vi "1.Main demo.vi"() -> ()   [LabVIEW 2010]
uses:
  UnderAutomation.Fanuc/UnderAutomation.Fanuc.lvlib
  C:/Users/fg/Documents/Fanuc.vi/LabVIEW_2024/UnderAutomation.Fanuc/lib/UnderAutomation.Fanuc.dll
  LabVIEW_2024/UnderAutomation.Fanuc/lib/UnderAutomation.Fanuc.dll
panel:
  out "CGTP Enabled":bool
  out "Cgtp":refnum<k24>
  out "SNPX connected":bool
  out "FTP connected":bool
  out "Telnet connected":bool
  in  "Tab Control":T1(tab)
  in  "HTTP Password":string caption="HTTP password"
  in  "HTTP Login":string caption="HTTP login (optional)"
  in  "Use CGTP":bool
  in  "Disconnect":bool
  in  "Test":bool
  in  "Key":string
  in  "Licensee":string
  in  "Use SNPX":bool
  in  "FTP password":string
  in  "FTP user":string
  in  "Use FTP":bool
  in  "Connect":bool
  in  "Telnet password":string
  in  "Use Telnet":bool
  in  "ConnectRoboguide":bool
  in  "RoboguideRobotPath":path caption="Path to \"Robot\" ROBOGUIDE folder that contains services.txt"
  in  "IP":string caption="Robot IP Address"
  out "License state":string
  out "Connect error":string
  out "CGTP warning":string
  in  "Abort":bool
  in  "Pause":bool
  in  "Program name":string caption="Program name without extension"
  in  "Run":bool
  in  "Write variable as real":bool
  in  "New integer value":i32
  in  "New real value":dbl
  in  "String value":string
  in  "Variable name":string
  in  "Write variable as integer":bool
  in  "Read variable":bool
  in  "Write variable as string":bool
  in  "Unsimulate all":bool
  in  "Unsimulate":bool
  in  "Simulate":bool
  in  "Set port value":bool
  in  "Variable set value":bool
  in  "Variable new value":string caption="New value"
  in  "Variable get value":bool
  in  "Variable name":string
  out "Telnet warning":string
  out "Current position":T2
  in  "Get current position":bool
  in  "Reset alarms":bool
  in  "Get task info":bool
  in  "Task name":string caption="Task name (program without extension)"
  in  "Abort all programs":bool
  in  "Clear variable":bool
  in  "Clear Program":bool
  in  "Hold":bool
  in  "Continue":bool
  in  "Abort":bool
  in  "Pause":bool
  in  "Program name":string caption="Program name without extension"
  in  "Run":bool
  out "TelnetError":string caption="Error :"
  out "TelnetSucceed":bool caption="Succeeded"
  out "KclCommand":string caption="Last command :"
  out "TaskInfo":T3
  out "Variable value":string
  in  "port":i32(ring) items=["DIN", "DOUT", "RDO", "OPOUT", "TPOUT", "WDI", "WDO", "AIN", "AOUT", "GIN", "GOUT"]
  in  "index":i32
  in  "value":i32
  out "FTP warning":string
  out "PosReg":T4(array[cluster])
  out "StrReg":string[](array[string])
  in  "Tab Control IO state":T5(tab)
  out "UI":cluster{"Id":i32, "Name":string, "Value":bool}[](array[cluster])
  out "UO":cluster{"Id":i32, "Name":string, "Value":bool}[](array[cluster])
  out "SI":cluster{"Id":i32, "Name":string, "Value":bool}[](array[cluster])
  out "SO":cluster{"Id":i32, "Name":string, "Value":bool}[](array[cluster])
  out "DIN":cluster{"Id":i32, "Name":string, "Value":bool}[](array[cluster])
  out "DOUT":cluster{"Id":i32, "Name":string, "Value":bool}[](array[cluster])
  out "RI":cluster{"Id":i32, "Name":string, "Value":bool}[](array[cluster])
  out "RO":cluster{"Id":i32, "Name":string, "Value":bool}[](array[cluster])
  out "FLG":cluster{"Id":i32, "Name":string, "Value":bool}[](array[cluster])
  in  "Tab Control position":enum32{"World", "Joints", "User frames"}(tab)
  out "World Positions":T6(array[cluster])
  out "JointsPosition":dbl[](array[numeric])
  out "UserFramePositions":T7(array[cluster])
  in  "Get current position":bool
  in  "Get IO State":bool
  in  "Port":i32(ring) items=["DIN", "DOUT", "UI", "UO", "SI", "SO", "RI", "RO", "FLG"]
  out "Errors":T8(array[cluster])
  in  "Get all errors":bool
  in  "Get safety status":bool
  out "SafetyStatus":T9
  out "NumReg":dbl[](array[numeric])
  in  "Get numeric registers":bool
  in  "Get string registers":bool
  in  "Get position registers":bool
  out "SNPX warning":string
  in  "Tab Control snpx register":enum32{"Cartesian", "Joints"}(tab)
  in  "Cartesian position 2":T10
  in  "Write cartesian position register":bool
  in  "Joints position":dbl[](array[numeric])
  in  "Write joints position register":bool
  in  "Position register":i32
  in  "Read position register":bool
  out "Value":string
  in  "New value":string
  in  "String register":i32
  in  "Read string register":bool
  in  "Write string register":bool
  in  "Continuous read world position":bool
  out "JointsPosition":dbl[](array[numeric])
  out "Cartesian position":T11
  out "UserTool":i16
  out "error out":errorcluster
  in  "Continuous read user frame position":bool
  in  "userFrame":i32
  out "Cartesian position":T11
  out "UserTool":i16
  out "error out 2":errorcluster
  in  "Numeric register":i32
  in  "New value":sgl
  out "Value":sgl
  in  "Read numeric register":bool
  in  "Write numeric register":bool
  out "UserFrame":i16
  out "UserTool":i16
  in  "stop":bool
  out "Snpx":refnum<k24>
  out "Ftp":refnum<k24>
  out "Telnet":refnum<k24>
  out "robot":refnum<k24>
  # "UnderAutomation"
  # "https://underautomation.com/fanuc"
  # "+"
  # "LabVIEW demo app for remote control and monitoring of your Fanuc robot"
  # "Connect to robot"
  # "2. Ensure you have a trial or lifetime valid license"
  # "1. Set Fanuc robot address"
  # "This is a commercial library, you have a 30-day trial period. But you can use it forever if you buy a perpetual licence for your company (regardless of the number of robot, applications or developers)."
  # "Connect to real robot"
  # "Connect to ROBOGUIDE"
  # "If you have a license :"
  # "3. Select the services you want to connect to"
  # "CGTP"
  # "Telnet"
  # "FTP"
  # "SNPX"
  # "You need option R553 \"HMI Device SNPX\" \nor R651 FRL"
  # "How to enable Telnet : https://underautomation.com/fanuc/documentation/enable-telnet"
  # "See : https://underautomation.com/fanuc/documentation/snpx"
  # "4. Connect to the robot"
  # "CGTP"
  # "Please note that other CGTP features are available and can be provided upon request. Please contact UnderAutomation."
  # "Program execution"
  # "Variable"
  # "Telnet"
  # "Variables"
  # "Program execution"
  # "Task"
  # "Ports"
  # "Current position"
  # "Alarms"
  # "FTP"
  # "Current Position"
  # "IO State"
  # "Errors"
  # "Registers"
  # "Safety status"
  # "SNPX"
  # "Numeric registers"
  # "String registers"
  # "Read world position"
  # "Read user frame position"
  # "Position registers"
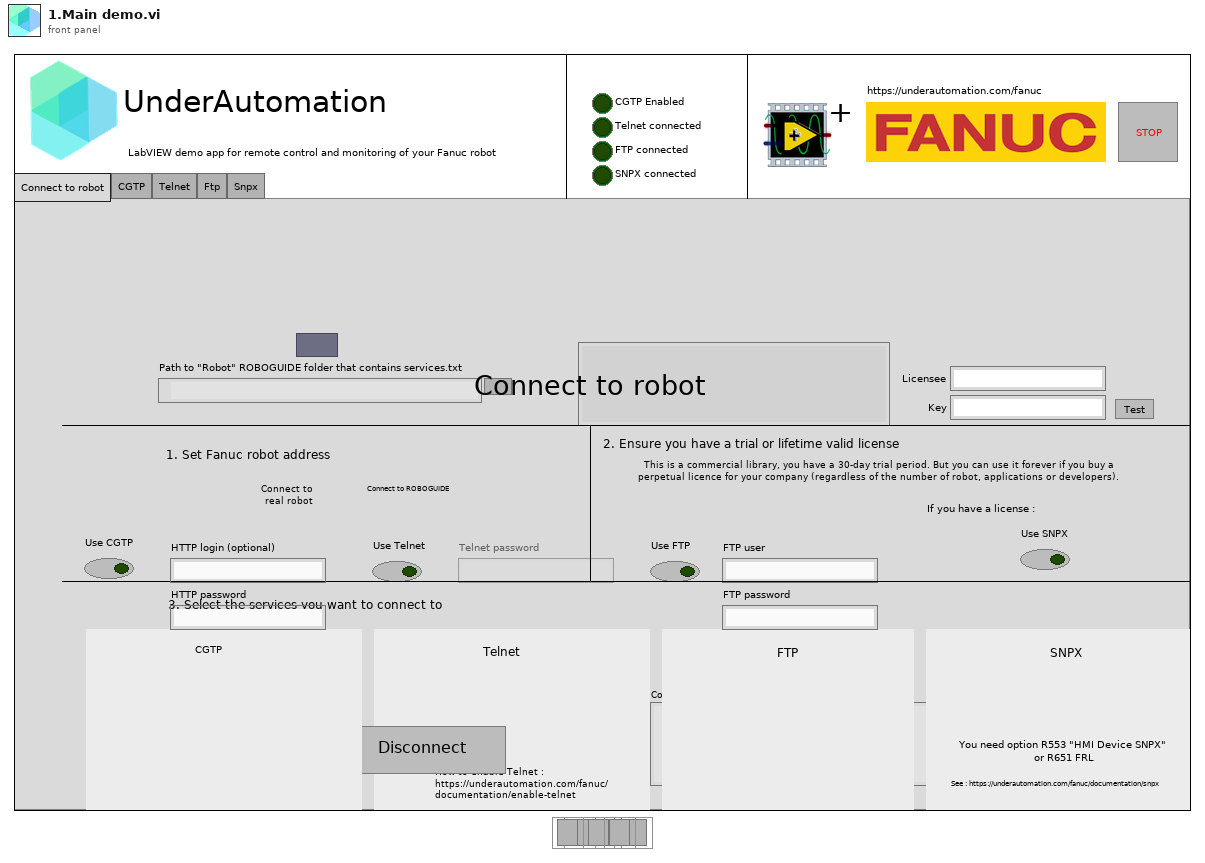
[diagram p1: front panel]
types:
  T1 = enum32{"Connect to robot", "CGTP", "Telnet", "Ftp", "Snpx"}
  T2 = cluster{"X":dbl, "Y":dbl, "Z":dbl, "W":dbl, "P":dbl, "R":dbl}
  T3 = cluster{"CurrentLine":i32, "RoutineName":string, "SystemTask":bool, "TaskName":string, "TaskNumber":i32, "TaskStatus":i32, "TaskStatusStr":string}
  T4 = cluster{"X":dbl, "Y":dbl, "Z":dbl, "W":dbl, "P":dbl, "R":dbl}[][]
  T5 = enum32{"UI", "UO", "SI", "SO", "DIN", "DOUT", "RI", "RO", "FLG"}
  T6 = cluster{"Tool":i32, "Cartesian position":cluster{cluster{"ArmFrontBack":i32, "ArmLeftRight":i32, "ArmUpDown":i32, "TurnAxis1":i32, "TurnAxis2":i32, "TurnAxis3":i32, "WristFlip":i32}, "X":dbl, "Y":dbl, "Z":dbl, "W":dbl, "P":dbl, "R":dbl}}[]
  T7 = cluster{"Frame":i32, "Tool":i32, "Cartesian position":cluster{cluster{"ArmFrontBack":i32, "ArmLeftRight":i32, "ArmUpDown":i32, "TurnAxis1":i32, "TurnAxis2":i32, "TurnAxis3":i32, "WristFlip":i32}, "X":dbl, "Y":dbl, "Z":dbl, "W":dbl, "P":dbl, "R":dbl}}[]
  T8 = cluster{"Id":i32, "IsReset":bool, "Text":string}[]
  T9 = cluster{"BeltBroken":bool, "ExternalEStop":bool, "FenceOpen":bool, "HandBroken":bool, "LowAirAlarm":bool, "NonTeacherEnb":bool, "OverTravel":bool, "SOPEStop":bool, "SVOFFDetect":bool, "TPDeadman":bool, "TPEnable":bool, "TPEStop":bool}
  T10 = cluster{"Configuration":cluster{"ArmFrontBack":i32, "ArmLeftRight":i32, "ArmUpDown":i32, "TurnAxis1":i32, "TurnAxis2":i32, "TurnAxis3":i32, "WristFlip":i32}, "X":dbl, "Y":dbl, "Z":dbl, "W":dbl, "P":dbl, "R":dbl}
  T11 = cluster{"Cartesian position":cluster{cluster{"ArmFrontBack":i32, "ArmLeftRight":i32, "ArmUpDown":i32, "TurnAxis1":i32, "TurnAxis2":i32, "TurnAxis3":i32, "WristFlip":i32}, "X":dbl, "Y":dbl, "Z":dbl, "W":dbl, "P":dbl, "R":dbl}, "Extension":cluster{"E1":dbl, "E2":dbl, "E3":dbl, "T4":i16, "T5":i16, "T6":i16}}
  T12 = enum8{"Enabled", "Disabled", "Disabled and Grayed Out"}
  T13 = cluster{"Id":i32, "Values":dbl[], "UserFramePositions":cluster{"Frame":i32, "Tool":i32, "Cartesian position":cluster{cluster{"ArmFrontBack":i32, "ArmLeftRight":i32, "ArmUpDown":i32, "TurnAxis1":i32, "TurnAxis2":i32, "TurnAxis3":i32, "WristFlip":i32}, "X":dbl, "Y":dbl, "Z":dbl, "W":dbl, "P":dbl, "R":dbl}}[], "World Positions":cluster{"Tool":i32, "Cartesian position":cluster{cluster{"ArmFrontBack":i32, "ArmLeftRight":i32, "ArmUpDown":i32, "TurnAxis1":i32, "TurnAxis2":i32, "TurnAxis3":i32, "WristFlip":i32}, "X":dbl, "Y":dbl, "Z":dbl, "W":dbl, "P":dbl, "R":dbl}}[]}[]
  T14 = cluster{"Id":i32, "Name":string, "Port":i32, "Value":bool, "PortStr":string}[]
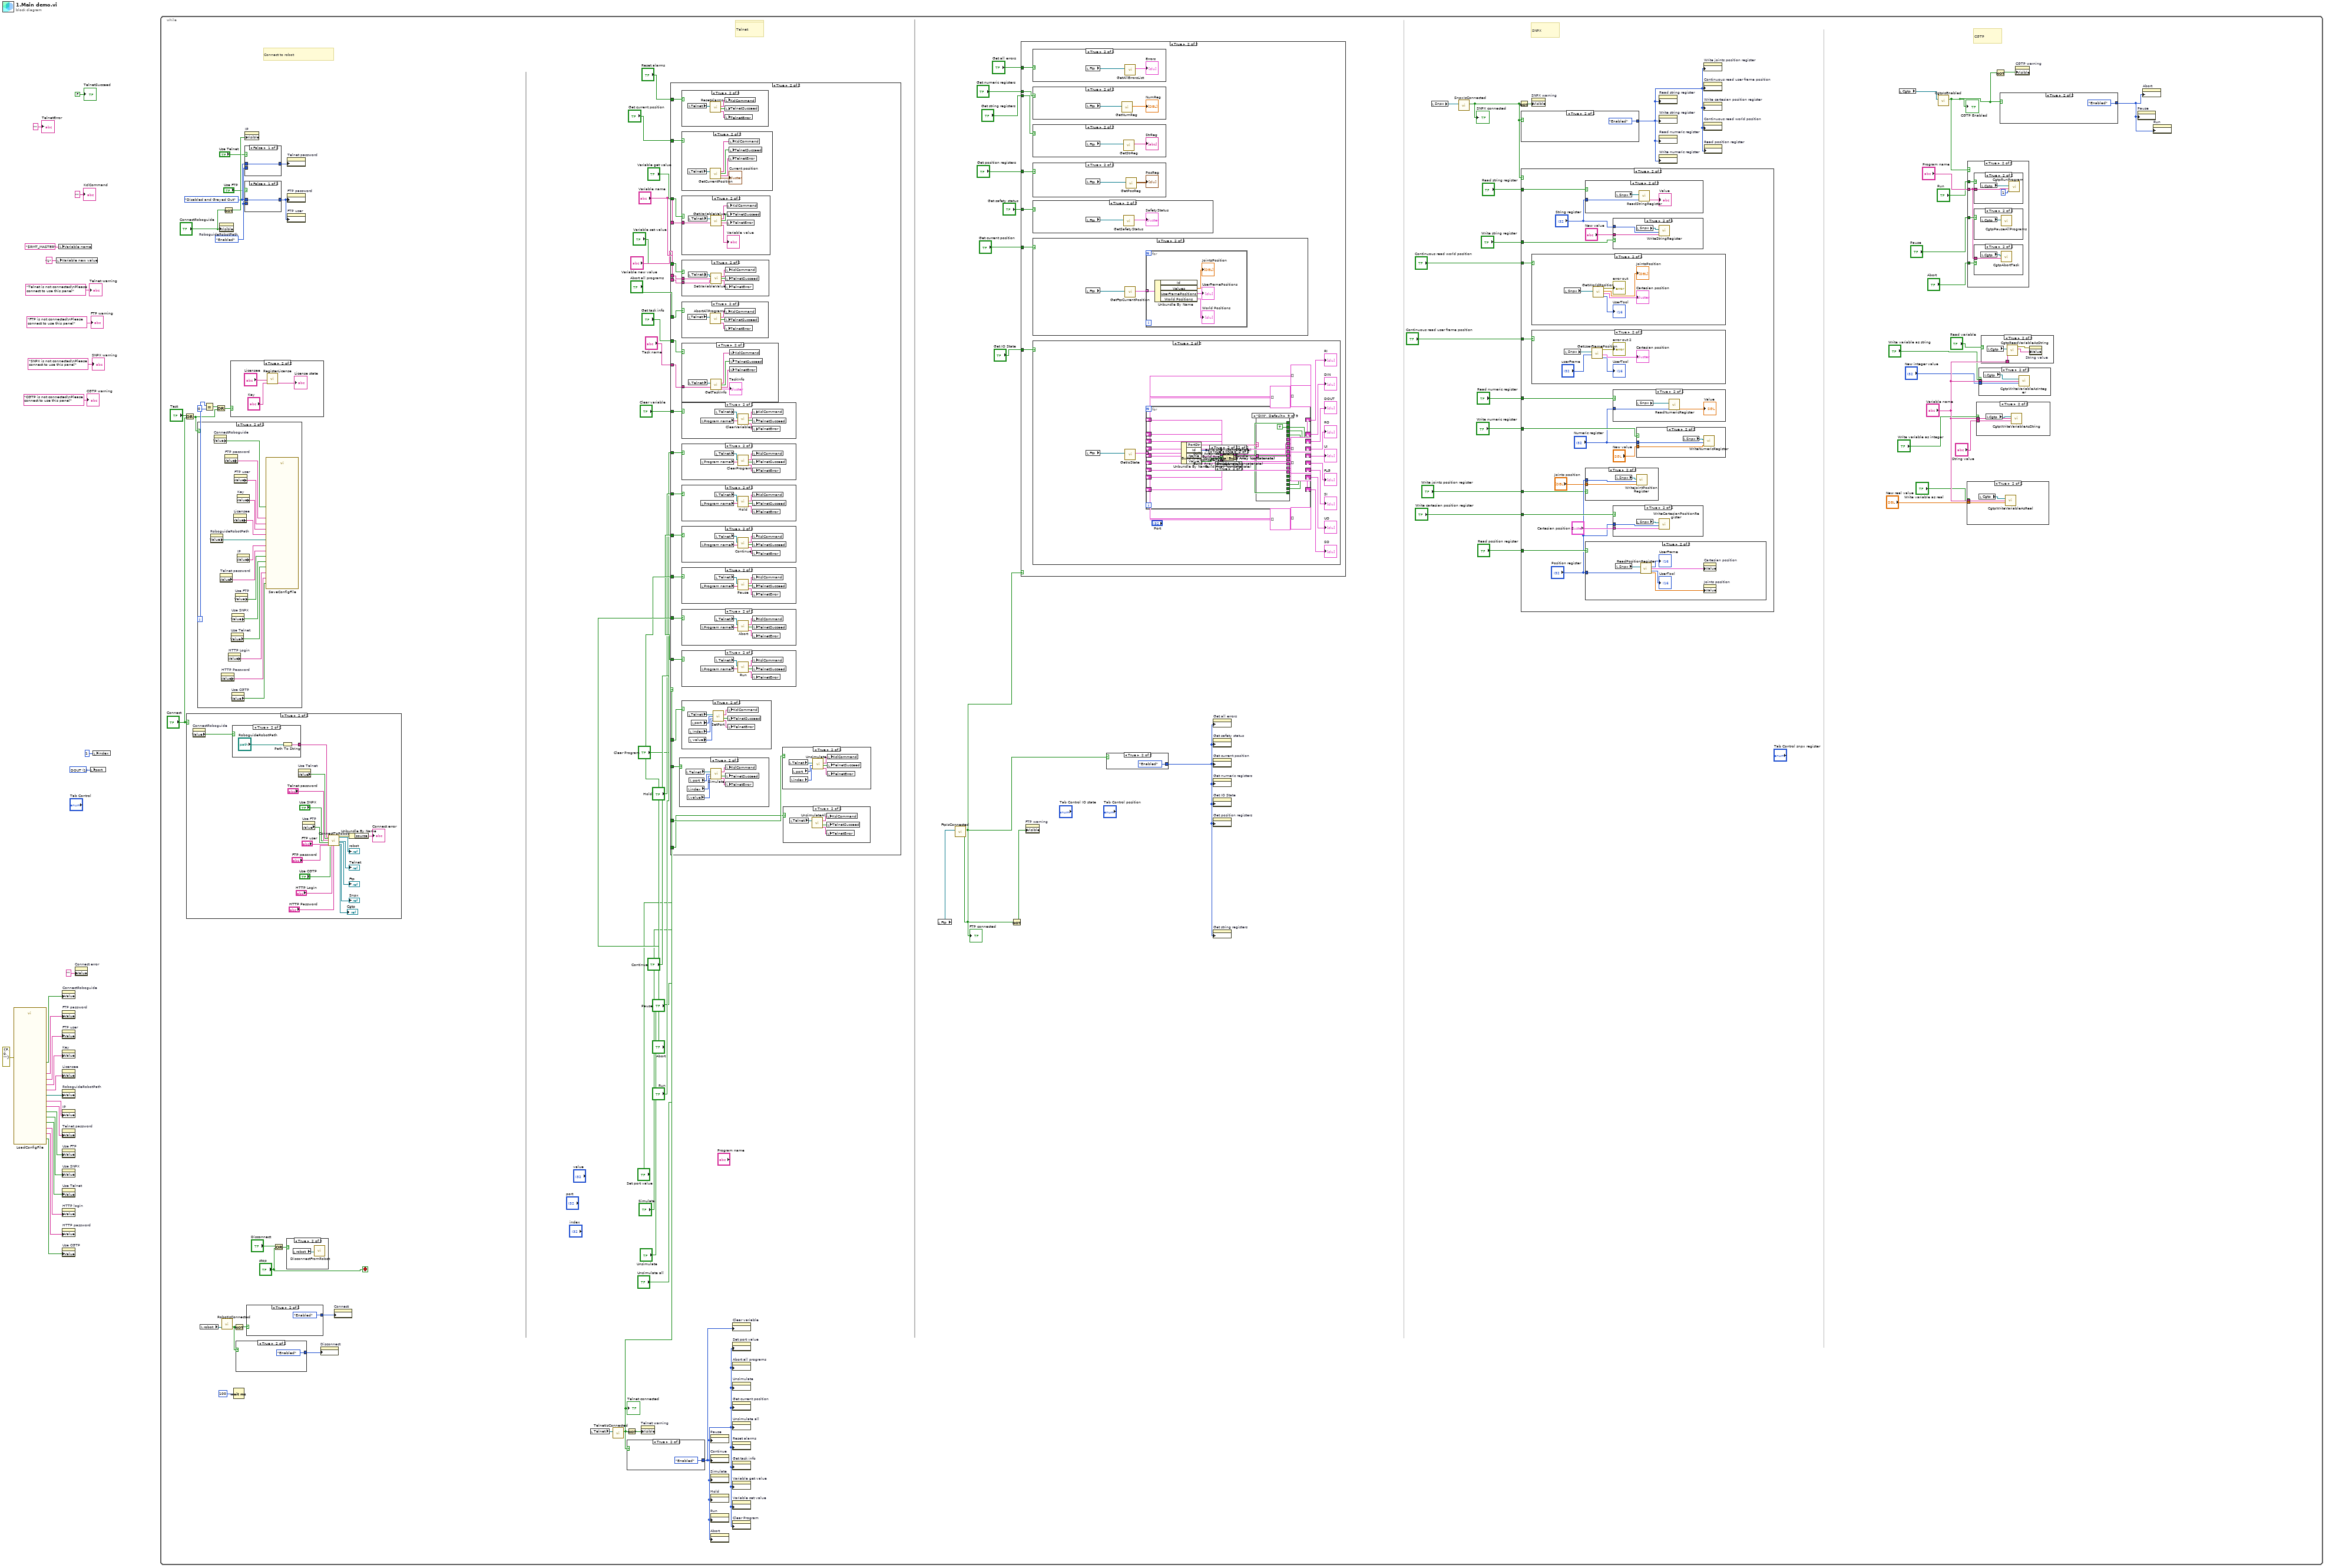
[diagram p0: block diagram]
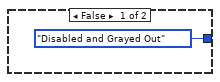
[diagram p10: hidden frame]
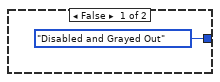
[diagram p11: hidden frame]
diagram:
  w7 = 1 items=["DIN", "DOUT", "RDO", "OPOUT", "TPOUT", "WDI", "WDO", "AIN", "AOUT", "GIN", "GOUT"] ("port")
  n1 = call "LoadConfigFile.vi"("error in (no error)"=errorcluster {"status"=FALSE, "code"=0, "source"=""}) -> ("Use CGTP"=w2:bool, "HTTP login"=w3:string, "HTTP password"=w4:string, "FTP password"=w24:string, "Licensee"=w16:string, "FTP user"=w23:string, "Key"=w17:string, "Use FTP"=w20:bool, "IP"=w26:string, "RoboguideRobotPath"=w22:path, "ConnectRoboguide"=w25:bool, "Use Telnet"=w18:bool, "Telnet password"=w21:string, "Use SNPX"=w19:bool)  [unwired: 12 in, 1 out]
  n2 = local write "Variable new value"("1" ("Variable new value")) -> ()
  n3 = local write "Variable name"("$RMT_MASTER" ("Variable name")) -> ()
  n4 = property on="ConnectRoboguide" class="Bool (strict)"("Value"=w25) -> ()  [unwired: 2 in, 2 out]
  n5 = property on="FTP password" class="Str"("Value"=w24) -> ()  [unwired: 2 in, 2 out]
  n6 = property on="FTP user" class="Str"("Value"=w23) -> ()  [unwired: 2 in, 2 out]
  n7 = property on="Key" class="Str"("Value"=w17) -> ()  [unwired: 2 in, 2 out]
  n8 = property on="Licensee" class="Str"("Value"=w16) -> ()  [unwired: 2 in, 2 out]
  n9 = property on="RoboguideRobotPath" class="Path"("Value"=w22) -> ()  [unwired: 2 in, 2 out]
  n10 = property on="IP" class="Str"("Value"=w26) -> ()  [unwired: 2 in, 2 out]
  n11 = property on="Telnet password" class="Str"("Value"=w21) -> ()  [unwired: 2 in, 2 out]
  n12 = property on="Use FTP" class="Bool (strict)"("Value"=w20) -> ()  [unwired: 2 in, 2 out]
  n13 = property on="Use SNPX" class="Bool (strict)"("Value"=w19) -> ()  [unwired: 2 in, 2 out]
  n14 = property on="Use Telnet" class="Bool (strict)"("Value"=w18) -> ()  [unwired: 2 in, 2 out]
  n15 = property on="HTTP login" class="Str"("Value"=w3) -> ()  [unwired: 2 in, 2 out]
  n16 = property on="HTTP password" class="Str"("Value"=w4) -> ()  [unwired: 2 in, 2 out]
  n17 = property on="Use CGTP" class="Bool (strict)"("Value"=w2) -> ()  [unwired: 2 in, 2 out]
  n18 = property on="Connect error" class="Str"("Value"="" ("Connect error")) -> ()  [unwired: 2 in, 2 out]
  n19 = local write "port"(w7) -> ()
  n20 = local write "index"(1 ("index")) -> ()
  n21 = while {
    i -> [w110]
    stop <- "stop" stop-if-true
    w102 = T12."Enabled" ("Disabled")
    w103 = T12."Disabled and Grayed Out" ("Disabled")
    # "CGTP"
    # "SNPX"
    # "FTP"
    # "Telnet"
    # "Connect to robot"
    n22 = Or(x="Test", y="Connect") -> (x .or. y?=w107:bool)
    n23 = case shown="True" "Connect" {
      frame False {
      }
      frame True {
        n24 = property on="ConnectRoboguide" class="Bool (strict)"() -> ("Value"=w490:bool)  [unwired: 2 in, 2 out]
        n25 = case shown="True" w490 {
          tunnel: ["IP" w492] -> w489
          frame False {
          }
          frame True {
            n26 = Path To String(path="RoboguideRobotPath") -> (string=w492:string)
          }
        }
        n27 = property on="Use Telnet" class="Bool (strict)"() -> ("Value"=w485:bool)  [unwired: 2 in, 2 out]
        n28 = property on="Use FTP" class="Bool (strict)"() -> ("Value"=w484:bool)  [unwired: 2 in, 2 out]
        n29 = call "ConnectToRobot.vi"("address"=w489, "Telnet enable"=w485, "Telnet KCL password"="Telnet password", "SNPX enable"="Use SNPX", "FTP enable"=w484, "FTP user"="FTP user", "FTP password"="FTP password", "CGTP enable"="Use CGTP", "HTTP login"="HTTP Login", "HTTP password"="HTTP Password") -> ("error out"=w483:errorcluster, "robot"=→"robot":refnum<k24>, "Telnet"=→"Telnet":refnum<k24>, "Ftp"=→"Ftp":refnum<k24>, "Snpx"=→"Snpx":refnum<k24>, "Cgtp"=→"Cgtp":refnum<k24>)  [unwired: 12 in]
        n30 = Unbundle By Name(w483) -> ("source"=→"Connect error":string)
      }
    }
    n31 = case shown="True" w107 {
      frame False {
      }
      frame True {
        n32 = property on="RoboguideRobotPath" class="Path"() -> ("Value"=w467:path)  [unwired: 2 in, 2 out]
        n33 = property on="ConnectRoboguide" class="Bool (strict)"() -> ("Value"=w472:bool)  [unwired: 2 in, 2 out]
        n34 = property on="Telnet password" class="Str"() -> ("Value"=w465:string)  [unwired: 2 in, 2 out]
        n35 = property on="HTTP Password" class="Str"() -> ("Value"=w459:string)  [unwired: 2 in, 2 out]
        n36 = property on="FTP password" class="Str"() -> ("Value"=w471:string)  [unwired: 2 in, 2 out]
        n37 = property on="HTTP Login" class="Str"() -> ("Value"=w460:string)  [unwired: 2 in, 2 out]
        n38 = property on="Use Telnet" class="Bool (strict)"() -> ("Value"=w462:bool)  [unwired: 2 in, 2 out]
        n39 = property on="Use SNPX" class="Bool (strict)"() -> ("Value"=w463:bool)  [unwired: 2 in, 2 out]
        n40 = property on="Use CGTP" class="Bool (strict)"() -> ("Value"=w461:bool)  [unwired: 2 in, 2 out]
        n41 = property on="Licensee" class="Str"() -> ("Value"=w468:string)  [unwired: 2 in, 2 out]
        n42 = property on="FTP user" class="Str"() -> ("Value"=w470:string)  [unwired: 2 in, 2 out]
        n43 = property on="Use FTP" class="Bool (strict)"() -> ("Value"=w464:bool)  [unwired: 2 in, 2 out]
        n44 = property on="Key" class="Str"() -> ("Value"=w469:string)  [unwired: 2 in, 2 out]
        n45 = property on="IP" class="Str"() -> ("Value"=w466:string)  [unwired: 2 in, 2 out]
        n46 = call "SaveConfigFile.vi"("IP"=w466, "RoboguideRobotPath"=w467, "ConnectRoboguide"=w472, "Use Telnet"=w462, "Telnet password"=w465, "Use FTP"=w464, "FTP user"=w470, "FTP password"=w471, "Use SNPX"=w463, "Licensee"=w468, "Use CGTP"=w461, "Key"=w469, "HTTP Login"=w460, "HTTP Password"=w459) -> ()  [unwired: 14 in]
      }
    }
    n47 = local read "robot"() -> (w77:refnum<k24>)
    n48 = Equal?(x=w110, y=0) -> (x = y?=w108:bool)
    n49 = Or(x=w108, y=w107) -> (x .or. y?=w106:bool)
    n50 = property on="RoboguideRobotPath" class="Path"("Visible"="ConnectRoboguide") -> ()  [unwired: 2 in, 2 out]
    n51 = call "RobotIsConnected.vi"("robot"=w77) -> ("Connected"=w75:bool)  [unwired: 1 in, 1 out]
    n52 = Not(x="ConnectRoboguide") -> (.not. x?=w114:bool)
    n53 = case shown="True" w106 {
      frame False {
      }
      frame True {
        n54 = call "RegisterLicense.vi"("key"="Key", "licensee"="Licensee") -> ("status"=→"License state":string)  [unwired: 7 in, 2 out]
      }
    }
    n55 = Wait (ms)(milliseconds to wait=u32 100) -> ()  [unwired: 1 out]
    n56 = Not(x=w75) -> (.not. x?=w76:bool)
    n57 = case shown="True" w75 {
      tunnel: [T12."Disabled and Grayed Out" ("Disabled") T12."Enabled" ("Disabled")] -> w74
      frame False {
      }
      frame True {
      }
    }
    n58 = property on="IP" class="Str"("Visible"=w114) -> ()  [unwired: 2 in, 2 out]
    n59 = case shown="False" "Use Telnet" {
      tunnel: w102 -> [_ w455]
      tunnel: [w454 w455] -> w104
      tunnel: w103 -> [w454 _]
      frame False {
      }
      frame True {
      }
    }
    n60 = case shown="False" "Use FTP" {
      tunnel: w102 -> [_ w453]
      tunnel: [w452 w453] -> w100
      tunnel: w103 -> [w452 _]
      frame False {
      }
      frame True {
      }
    }
    n61 = case shown="True" w76 {
      tunnel: [T12."Disabled and Grayed Out" ("Disabled") T12."Enabled" ("Disabled")] -> w73
      frame False {
      }
      frame True {
      }
    }
    n62 = Or(x="Disconnect", y="stop") -> (x .or. y?=w79:bool)
    n63 = case shown="True" w79 {
      frame False {
      }
      frame True {
        n64 = local read "robot"() -> (w338:refnum<k24>)
        n65 = call "DisconnectFromRobot.vi"("robot"=w338) -> ()  [unwired: 26 in, 1 out]
      }
    }
    n66 = property on="Telnet password" class="Str"("DisabledEnum"=w104) -> ()  [unwired: 2 in, 2 out]
    n67 = property on="FTP password" class="Str"("DisabledEnum"=w100) -> ()  [unwired: 2 in, 2 out]
    n68 = property on="FTP user" class="Str"("DisabledEnum"=w100) -> ()  [unwired: 2 in, 2 out]
    n69 = property on="Disconnect" class="Bool"("DisabledEnum"=w74) -> ()  [unwired: 2 in, 2 out]
    n70 = property on="Connect" class="Bool"("DisabledEnum"=w73) -> ()  [unwired: 2 in, 2 out]
    n71 = local read "Telnet"() -> (w99:refnum<k24>)
    n72 = call "TelnetIsConnected.vi"("Telnet"=w99) -> ("Connected"=w97:bool)  [unwired: 9 in, 1 out]
    "Telnet connected" <- w97
    n73 = Not(x=w97) -> (.not. x?=w96:bool)
    n74 = case shown="True" w97 {
      tunnel: [T12."Disabled and Grayed Out" ("Disabled") T12."Enabled" ("Disabled")] -> w68
      frame False {
      }
      frame True {
      }
    }
    n75 = property on="Telnet warning" class="Str"("Visible"=w96) -> ()  [unwired: 2 in, 2 out]
    n76 = case shown="True" w97 {
      tunnel: "Run" -> [_ w361]
      tunnel: "Abort" -> [_ w360]
      tunnel: "Pause" -> [_ w359]
      tunnel: "Continue" -> [_ w358]
      tunnel: "Hold" -> [_ w357]
      tunnel: "Clear variable" -> [_ w356]
      tunnel: "Clear Program" -> [_ w355]
      tunnel: "Abort all programs" -> [_ w354]
      tunnel: "Task name" -> [_ w353]
      tunnel: "Get task info" -> [_ w352]
      tunnel: "Reset alarms" -> [_ w351]
      tunnel: "Get current position" -> [_ w350]
      tunnel: "Variable get value" -> [_ w349]
      tunnel: "Variable name" -> [_ w348]
      tunnel: "Variable name" -> [_ w347]
      tunnel: "Variable new value" -> [_ w346]
      tunnel: "Variable set value" -> [_ w345]
      tunnel: "Set port value" -> [_ w344]
      tunnel: "Simulate" -> [_ w343]
      tunnel: "Unsimulate" -> [_ w342]
      tunnel: "Unsimulate all" -> [_ w341]
      frame False {
      }
      frame True {
        n77 = case shown="True" w343 {
          frame False {
          }
          frame True {
            n78 = local read "Telnet"() -> (w375:refnum<k24>)
            n79 = local read "index"() -> (w372:i32)
            n80 = local read "value"() -> (w374:i32)
            n81 = local read "port"() -> (w373:i32)
            n82 = call "Simulate.vi"("Telnet"=w375, "port"=w373, "index"=w372, "value"=w374) -> ("KclCommand"=w378:string, "Succeed"=w377:bool, "ErrorText"=w376:string)  [unwired: 8 in, 1 out]
            n83 = local write "KclCommand"(w378) -> ()
            n84 = local write "TelnetSucceed"(w377) -> ()
            n85 = local write "TelnetError"(w376) -> ()
          }
        }
        n86 = case shown="True" w351 {
          frame False {
          }
          frame True {
            n87 = local read "Telnet"() -> (w406:refnum<k24>)
            n88 = call "ResetAlarms.vi"("Telnet"=w406) -> ("ErrorText"=w404:string, "Succeed"=w405:bool, "KclCommand"=w403:string)  [unwired: 7 in, 1 out]
            n89 = local write "KclCommand"(w403) -> ()
            n90 = local write "TelnetSucceed"(w405) -> ()
            n91 = local write "TelnetError"(w404) -> ()
          }
        }
        n92 = case shown="True" w350 {
          frame False {
          }
          frame True {
            n93 = local read "Telnet"() -> (w402:refnum<k24>)
            n94 = call "GetCurrentPosition.vi"("Telnet"=w402) -> ("KclCommand"=w400:string, "Succeed"=w399:bool, "ErrorText"=w398:string, "Position"=→"Current position":T2)  [unwired: 10 in, 1 out]
            n95 = local write "KclCommand"(w400) -> ()
            n96 = local write "TelnetSucceed"(w399) -> ()
            n97 = local write "TelnetError"(w398) -> ()
          }
        }
        n98 = case shown="True" w349 {
          tunnel: w348 -> [_ w396]
          frame False {
          }
          frame True {
            n99 = local read "Telnet"() -> (w397:refnum<k24>)
            n100 = call "GetVariableValue.vi"("Telnet"=w397, "name"=w396) -> ("KclCommand"=w392:string, "Succeed"=w393:bool, "ErrorText"=w394:string, "RawValue"=→"Variable value":string)  [unwired: 9 in, 1 out]
            n101 = local write "KclCommand"(w392) -> ()
            n102 = local write "TelnetSucceed"(w393) -> ()
            n103 = local write "TelnetError"(w394) -> ()
          }
        }
        n104 = case shown="True" w345 {
          tunnel: w347 -> [_ w390]
          tunnel: w346 -> [_ w389]
          frame False {
          }
          frame True {
            n105 = local read "Telnet"() -> (w391:refnum<k24>)
            n106 = call "SetVariableValue.vi"("Telnet"=w391, "value"=w389, "name"=w390) -> ("KclCommand"=w388:string, "Succeed"=w387:bool, "ErrorText"=w386:string)  [unwired: 9 in, 1 out]
            n107 = local write "KclCommand"(w388) -> ()
            n108 = local write "TelnetSucceed"(w387) -> ()
            n109 = local write "TelnetError"(w386) -> ()
          }
        }
        n110 = case shown="True" w354 {
          frame False {
          }
          frame True {
            n111 = local read "Telnet"() -> (w413:refnum<k24>)
            n112 = call "AbortAllPrograms.vi"("Telnet"=w413) -> ("ErrorText"=w414:string, "Succeed"=w415:bool, "KclCommand"=w416:string)  [unwired: 7 in, 1 out]
            n113 = local write "KclCommand"(w416) -> ()
            n114 = local write "TelnetSucceed"(w415) -> ()
            n115 = local write "TelnetError"(w414) -> ()
          }
        }
        n116 = case shown="True" w352 {
          tunnel: w353 -> [_ w411]
          frame False {
          }
          frame True {
            n117 = local read "Telnet"() -> (w412:refnum<k24>)
            n118 = call "GetTaskInfo.vi"("Telnet"=w412, "task"=w411) -> ("KclCommand"=w409:string, "Succeed"=w408:bool, "ErrorText"=w407:string, "TaskInfo"=→"TaskInfo":T3)  [unwired: 9 in, 1 out]
            n119 = local write "KclCommand"(w409) -> ()
            n120 = local write "TelnetSucceed"(w408) -> ()
            n121 = local write "TelnetError"(w407) -> ()
          }
        }
        n122 = case shown="True" w356 {
          frame False {
          }
          frame True {
            n123 = local read "Program name"() -> (w417:string)
            n124 = local read "Telnet"() -> (w418:refnum<k24>)
            n125 = call "ClearVariables.vi"("program"=w417, "Telnet"=w418) -> ("ErrorText"=w419:string, "Succeed"=w420:bool, "KclCommand"=w421:string)  [unwired: 6 in, 1 out]
            n126 = local write "KclCommand"(w421) -> ()
            n127 = local write "TelnetSucceed"(w420) -> ()
            n128 = local write "TelnetError"(w419) -> ()
          }
        }
        n129 = case shown="True" w355 {
          frame False {
          }
          frame True {
            n130 = local read "Program name"() -> (w422:string)
            n131 = local read "Telnet"() -> (w423:refnum<k24>)
            n132 = call "ClearProgram.vi"("program"=w422, "Telnet"=w423) -> ("ErrorText"=w424:string, "Succeed"=w425:bool, "KclCommand"=w426:string)  [unwired: 6 in, 1 out]
            n133 = local write "KclCommand"(w426) -> ()
            n134 = local write "TelnetSucceed"(w425) -> ()
            n135 = local write "TelnetError"(w424) -> ()
          }
        }
        n136 = case shown="True" w357 {
          frame False {
          }
          frame True {
            n137 = local read "Program name"() -> (w427:string)
            n138 = local read "Telnet"() -> (w428:refnum<k24>)
            n139 = call "Hold.vi"("program"=w427, "Telnet"=w428) -> ("ErrorText"=w429:string, "Succeed"=w430:bool, "KclCommand"=w431:string)  [unwired: 6 in, 1 out]
            n140 = local write "KclCommand"(w431) -> ()
            n141 = local write "TelnetSucceed"(w430) -> ()
            n142 = local write "TelnetError"(w429) -> ()
          }
        }
        n143 = case shown="True" w358 {
          frame False {
          }
          frame True {
            n144 = local read "Program name"() -> (w432:string)
            n145 = local read "Telnet"() -> (w433:refnum<k24>)
            n146 = call "Continue.vi"("program"=w432, "Telnet"=w433) -> ("ErrorText"=w434:string, "Succeed"=w435:bool, "KclCommand"=w436:string)  [unwired: 6 in, 1 out]
            n147 = local write "KclCommand"(w436) -> ()
            n148 = local write "TelnetSucceed"(w435) -> ()
            n149 = local write "TelnetError"(w434) -> ()
          }
        }
        n150 = case shown="True" w359 {
          frame False {
          }
          frame True {
            n151 = local read "Program name"() -> (w437:string)
            n152 = local read "Telnet"() -> (w438:refnum<k24>)
            n153 = call "Pause.vi"("program"=w437, "Telnet"=w438) -> ("ErrorText"=w439:string, "Succeed"=w440:bool, "KclCommand"=w441:string)  [unwired: 6 in, 1 out]
            n154 = local write "KclCommand"(w441) -> ()
            n155 = local write "TelnetSucceed"(w440) -> ()
            n156 = local write "TelnetError"(w439) -> ()
          }
        }
        n157 = case shown="True" w360 {
          frame False {
          }
          frame True {
            n158 = local read "Program name"() -> (w442:string)
            n159 = local read "Telnet"() -> (w443:refnum<k24>)
            n160 = call "Abort.vi"("program"=w442, "Telnet"=w443) -> ("ErrorText"=w444:string, "Succeed"=w445:bool, "KclCommand"=w446:string)  [unwired: 6 in, 1 out]
            n161 = local write "KclCommand"(w446) -> ()
            n162 = local write "TelnetSucceed"(w445) -> ()
            n163 = local write "TelnetError"(w444) -> ()
          }
        }
        n164 = case shown="True" w361 {
          frame False {
          }
          frame True {
            n165 = local read "Program name"() -> (w447:string)
            n166 = local read "Telnet"() -> (w448:refnum<k24>)
            n167 = call "Run.vi"("program"=w447, "Telnet"=w448) -> ("ErrorText"=w449:string, "Succeed"=w450:bool, "KclCommand"=w451:string)  [unwired: 6 in, 1 out]
            n168 = local write "KclCommand"(w451) -> ()
            n169 = local write "TelnetSucceed"(w450) -> ()
            n170 = local write "TelnetError"(w449) -> ()
          }
        }
        n171 = case shown="True" w344 {
          frame False {
          }
          frame True {
            n172 = local read "Telnet"() -> (w382:refnum<k24>)
            n173 = local read "index"() -> (w379:i32)
            n174 = local read "value"() -> (w381:i32)
            n175 = local read "port"() -> (w380:i32)
            n176 = call "SetPort.vi"("Telnet"=w382, "port"=w380, "index"=w379, "value"=w381) -> ("KclCommand"=w385:string, "Succeed"=w384:bool, "ErrorText"=w383:string)  [unwired: 8 in, 1 out]
            n177 = local write "KclCommand"(w385) -> ()
            n178 = local write "TelnetSucceed"(w384) -> ()
            n179 = local write "TelnetError"(w383) -> ()
          }
        }
        n180 = case shown="True" w342 {
          frame False {
          }
          frame True {
            n181 = local read "Telnet"() -> (w368:refnum<k24>)
            n182 = local read "index"() -> (w366:i32)
            n183 = local read "port"() -> (w367:i32)
            n184 = call "Unsimulate.vi"("index"=w366, "port"=w367, "Telnet"=w368) -> ("ErrorText"=w369:string, "Succeed"=w370:bool, "KclCommand"=w371:string)  [unwired: 5 in, 1 out]
            n185 = local write "KclCommand"(w371) -> ()
            n186 = local write "TelnetSucceed"(w370) -> ()
            n187 = local write "TelnetError"(w369) -> ()
          }
        }
        n188 = case shown="True" w341 {
          frame False {
          }
          frame True {
            n189 = local read "Telnet"() -> (w362:refnum<k24>)
            n190 = call "UnsimulateAll.vi"("Telnet"=w362) -> ("KclCommand"=w365:string, "Succeed"=w364:bool, "ErrorText"=w363:string)  [unwired: 11 in, 1 out]
            n191 = local write "KclCommand"(w365) -> ()
            n192 = local write "TelnetSucceed"(w364) -> ()
            n193 = local write "TelnetError"(w363) -> ()
          }
        }
      }
    }
    n194 = property on="Pause" class="Bool"("DisabledEnum"=w68) -> ()  [unwired: 2 in, 2 out]
    n195 = property on="Continue" class="Bool"("DisabledEnum"=w68) -> ()  [unwired: 2 in, 2 out]
    n196 = property on="Simulate" class="Bool"("DisabledEnum"=w68) -> ()  [unwired: 2 in, 2 out]
    n197 = property on="Hold" class="Bool"("DisabledEnum"=w68) -> ()  [unwired: 2 in, 2 out]
    n198 = property on="Run" class="Bool"("DisabledEnum"=w68) -> ()  [unwired: 2 in, 2 out]
    n199 = property on="Abort" class="Bool"("DisabledEnum"=w68) -> ()  [unwired: 2 in, 2 out]
    n200 = property on="Clear variable" class="Bool"("DisabledEnum"=w68) -> ()  [unwired: 2 in, 2 out]
    n201 = property on="Set port value" class="Bool"("DisabledEnum"=w68) -> ()  [unwired: 2 in, 2 out]
    n202 = property on="Abort all programs" class="Bool"("DisabledEnum"=w68) -> ()  [unwired: 2 in, 2 out]
    n203 = property on="Unsimulate" class="Bool"("DisabledEnum"=w68) -> ()  [unwired: 2 in, 2 out]
    n204 = property on="Get current position" class="Bool"("DisabledEnum"=w68) -> ()  [unwired: 2 in, 2 out]
    n205 = property on="Unsimulate all" class="Bool"("DisabledEnum"=w68) -> ()  [unwired: 2 in, 2 out]
    n206 = property on="Reset alarms" class="Bool"("DisabledEnum"=w68) -> ()  [unwired: 2 in, 2 out]
    n207 = property on="Get task info" class="Bool"("DisabledEnum"=w68) -> ()  [unwired: 2 in, 2 out]
    n208 = property on="Variable get value" class="Bool"("DisabledEnum"=w68) -> ()  [unwired: 2 in, 2 out]
    n209 = property on="Variable set value" class="Bool"("DisabledEnum"=w68) -> ()  [unwired: 2 in, 2 out]
    n210 = property on="Clear Program" class="Bool"("DisabledEnum"=w68) -> ()  [unwired: 2 in, 2 out]
    n211 = local read "Ftp"() -> (w67:refnum<k24>)
    n212 = call "FtpIsConnected.vi"("Ftp"=w67) -> ("Connected"=w58:bool)  [unwired: 9 in, 1 out]
    "FTP connected" <- w58
    n213 = Not(x=w58) -> (.not. x?=w59:bool)
    n214 = case shown="True" w58 {
      tunnel: "Get current position" -> [_ w201]
      tunnel: "Get IO State" -> [_ w200]
      tunnel: "Get all errors" -> [_ w199]
      tunnel: "Get safety status" -> [_ w198]
      tunnel: "Get numeric registers" -> [_ w197]
      tunnel: "Get string registers" -> [_ w196]
      tunnel: "Get position registers" -> [_ w195]
      frame False {
      }
      frame True {
        n215 = case shown="True" w199 {
          frame False {
          }
          frame True {
            n216 = local read "Ftp"() -> (w211:refnum<k24>)
            n217 = call "GetAllErrorsList.vi"("Ftp"=w211) -> ("Errors"=→"Errors":T8)  [unwired: 9 in, 1 out]
          }
        }
        n218 = case shown="True" w197 {
          frame False {
          }
          frame True {
            n219 = local read "Ftp"() -> (w207:refnum<k24>)
            n220 = call "GetNumReg.vi"("Ftp"=w207) -> ("NumReg"=→"NumReg":dbl[])  [unwired: 9 in, 1 out]
          }
        }
        n221 = case shown="True" w196 {
          frame False {
          }
          frame True {
            n222 = local read "Ftp"() -> (w205:refnum<k24>)
            n223 = call "GetStrReg.vi"("Ftp"=w205) -> ("StrReg"=→"StrReg":string[])  [unwired: 9 in, 1 out]
          }
        }
        n224 = case shown="True" w195 {
          frame False {
          }
          frame True {
            n225 = local read "Ftp"() -> (w203:refnum<k24>)
            n226 = call "GetPosReg.vi"("Ftp"=w203) -> ("PosReg"=→"PosReg":T4)  [unwired: 9 in, 1 out]
          }
        }
        n227 = case shown="True" w198 {
          frame False {
          }
          frame True {
            n228 = local read "Ftp"() -> (w209:refnum<k24>)
            n229 = call "GetSafetyStatus.vi"("Ftp"=w209) -> ("SafetyStatus"=→"SafetyStatus":T9)  [unwired: 9 in, 1 out]
          }
        }
        n230 = case shown="True" w201 {
          frame False {
          }
          frame True {
            n231 = local read "Ftp"() -> (w329:refnum<k24>)
            n232 = call "GetFtpCurrentPosition.vi"("Ftp"=w329) -> ("Current position"=w328:T13)  [unwired: 9 in, 1 out]
            n233 = for {
              tunnel: w328 -> [w332] mode=indexing
              n234 = Unbundle By Name(w332) -> ("Values"=→"JointsPosition":dbl[], "UserFramePositions"=→"UserFramePositions":T7, "World Positions"=→"World Positions":T6)  [unwired: 1 out]
            }
          }
        }
        n235 = case shown="True" w200 {
          frame False {
          }
          frame True {
            n236 = local read "Ftp"() -> (w231:refnum<k24>)
            n237 = call "GetIoState.vi"("Ftp"=w231) -> ("IO States"=w230:T14)  [unwired: 9 in, 1 out]
            n238 = for {
              tunnel: w230 -> [w273] mode=indexing
              shift-right: [w248] -> w229
              shift-left: cluster{"Id":i32, "Name":string, "Value":bool}[] [] ("Array") -> [w249]
              shift-right: [w246] -> w228
              shift-left: cluster{"Id":i32, "Name":string, "Value":bool}[] [] ("Array") -> [w247]
              shift-right: [w244] -> w221
              shift-left: cluster{"Id":i32, "Name":string, "Value":bool}[] [] ("Array") -> [w245]
              shift-right: [w242] -> w227
              shift-left: cluster{"Id":i32, "Name":string, "Value":bool}[] [] ("Array") -> [w243]
              shift-right: [w240] -> w226
              shift-left: cluster{"Id":i32, "Name":string, "Value":bool}[] [] ("Array") -> [w241]
              shift-right: [w238] -> w225
              shift-left: cluster{"Id":i32, "Name":string, "Value":bool}[] [] ("Array") -> [w239]
              shift-right: [w236] -> w224
              shift-left: cluster{"Id":i32, "Name":string, "Value":bool}[] [] ("Array") -> [w237]
              shift-right: [w234] -> w223
              shift-left: cluster{"Id":i32, "Name":string, "Value":bool}[] [] ("Array") -> [w235]
              shift-right: [w232] -> w222
              shift-left: cluster{"Id":i32, "Name":string, "Value":bool}[] [] ("Array") -> [w233]
              n239 = Unbundle By Name(w273) -> ("PortStr"=w261:string, "Id"=w272:i32, "Name"=w271:string, "Value"=w270:bool)
              n240 = Bundle("Id"=w272, "Name"=w271, "Value"=w270) -> (w268:cluster{"Id":i32, "Name":string, "Value":bool})  [unwired: 1 in]
              n241 = case shown="\"DIN\", Default" w261 {
                tunnel: [_ _ _ _ _ _ _ w325 _] -> w269
                tunnel: w268 -> [w311 w313 w315 w317 w319 w321 w323 w325 w327]
                tunnel: [_ _ _ _ _ _ w323 _ _] -> w267
                tunnel: [_ _ _ _ _ _ _ _ w327] -> w259
                tunnel: [w311 _ _ _ _ _ _ _ _] -> w266
                tunnel: [_ w313 _ _ _ _ _ _ _] -> w265
                tunnel: [_ _ w315 _ _ _ _ _ _] -> w264
                tunnel: [_ _ _ w317 _ _ _ _ _] -> w263
                tunnel: [_ _ _ _ w319 _ _ _ _] -> w262
                tunnel: [_ _ _ _ _ w321 _ _ _] -> w260
                tunnel: [_ _ TRUE _ _ _ _ _ _] -> w258
                tunnel: [_ _ _ TRUE _ _ _ _ _] -> w257
                tunnel: [_ _ _ _ TRUE _ _ _ _] -> w256
                tunnel: [_ _ _ _ _ TRUE _ _ _] -> w255
                tunnel: [_ _ _ _ _ _ TRUE _ _] -> w254
                tunnel: [_ _ _ _ _ _ _ TRUE _] -> w253
                tunnel: [_ _ _ _ _ _ _ _ TRUE] -> w252
                tunnel: [TRUE _ _ _ _ _ _ _ _] -> w251
                tunnel: [_ TRUE _ _ _ _ _ _ _] -> w250
                frame "DOUT" {
                }
                frame "UI" {
                }
                frame "UO" {
                }
                frame "SI" {
                }
                frame "SO" {
                }
                frame "RI" {
                }
                frame "RO" {
                }
                frame "FLG" {
                }
                frame "DIN", Default {
                }
              }
              n242 = case shown="True" w255 {
                tunnel: w233 -> [w274 w276]
                tunnel: w260 -> [_ w275]
                tunnel: [w274 w277] -> w232
                frame False {
                }
                frame True {
                  n243 = Build Array (concatenate)(w276, w275) -> (w277:cluster{"Id":i32, "Name":string, "Value":bool}[])
                }
              }
              n244 = case shown="True" w256 {
                tunnel: w235 -> [w278 w280]
                tunnel: w262 -> [_ w279]
                tunnel: [w278 w281] -> w234
                frame False {
                }
                frame True {
                  n245 = Build Array (concatenate)(w280, w279) -> (w281:cluster{"Id":i32, "Name":string, "Value":bool}[])
                }
              }
              n246 = case shown="True" w257 {
                tunnel: w237 -> [w282 w284]
                tunnel: w263 -> [_ w283]
                tunnel: [w282 w285] -> w236
                frame False {
                }
                frame True {
                  n247 = Build Array (concatenate)(w284, w283) -> (w285:cluster{"Id":i32, "Name":string, "Value":bool}[])
                }
              }
              n248 = case shown="True" w258 {
                tunnel: w239 -> [w286 w288]
                tunnel: w264 -> [_ w287]
                tunnel: [w286 w289] -> w238
                frame False {
                }
                frame True {
                  n249 = Build Array (concatenate)(w288, w287) -> (w289:cluster{"Id":i32, "Name":string, "Value":bool}[])
                }
              }
              n250 = case shown="True" w250 {
                tunnel: w241 -> [w290 w292]
                tunnel: w265 -> [_ w291]
                tunnel: [w290 w293] -> w240
                frame False {
                }
                frame True {
                  n251 = Build Array (concatenate)(w292, w291) -> (w293:cluster{"Id":i32, "Name":string, "Value":bool}[])
                }
              }
              n252 = case shown="True" w251 {
                tunnel: w243 -> [w294 w296]
                tunnel: w266 -> [_ w295]
                tunnel: [w294 w297] -> w242
                frame False {
                }
                frame True {
                  n253 = Build Array (concatenate)(w296, w295) -> (w297:cluster{"Id":i32, "Name":string, "Value":bool}[])
                }
              }
              n254 = case shown="True" w252 {
                tunnel: w245 -> [w298 w300]
                tunnel: w259 -> [_ w299]
                tunnel: [w298 w301] -> w244
                frame False {
                }
                frame True {
                  n255 = Build Array (concatenate)(w300, w299) -> (w301:cluster{"Id":i32, "Name":string, "Value":bool}[])
                }
              }
              n256 = case shown="True" w254 {
                tunnel: w247 -> [w302 w304]
                tunnel: w267 -> [_ w303]
                tunnel: [w302 w305] -> w246
                frame False {
                }
                frame True {
                  n257 = Build Array (concatenate)(w304, w303) -> (w305:cluster{"Id":i32, "Name":string, "Value":bool}[])
                }
              }
              n258 = case shown="True" w253 {
                tunnel: w249 -> [w306 w308]
                tunnel: w269 -> [_ w307]
                tunnel: [w306 w309] -> w248
                frame False {
                }
                frame True {
                  n259 = Build Array (concatenate)(w308, w307) -> (w309:cluster{"Id":i32, "Name":string, "Value":bool}[])
                }
              }
            }
            "FLG" <- w229
            "RO" <- w228
            "DIN" <- w221
            "DOUT" <- w227
            "UI" <- w226
            "UO" <- w225
            "SI" <- w224
            "SO" <- w223
            "RI" <- w222
          }
        }
      }
    }
    n260 = property on="FTP warning" class="Str"("Visible"=w59) -> ()  [unwired: 2 in, 2 out]
    n261 = case shown="True" w58 {
      tunnel: [T12."Disabled and Grayed Out" ("Disabled") T12."Enabled" ("Disabled")] -> w57
      frame False {
      }
      frame True {
      }
    }
    n262 = property on="Get all errors" class="Bool"("DisabledEnum"=w57) -> ()  [unwired: 2 in, 2 out]
    n263 = property on="Get safety status" class="Bool"("DisabledEnum"=w57) -> ()  [unwired: 2 in, 2 out]
    n264 = property on="Get current position" class="Bool"("DisabledEnum"=w57) -> ()  [unwired: 2 in, 2 out]
    n265 = property on="Get numeric registers" class="Bool"("DisabledEnum"=w57) -> ()  [unwired: 2 in, 2 out]
    n266 = property on="Get IO State" class="Bool"("DisabledEnum"=w57) -> ()  [unwired: 2 in, 2 out]
    n267 = property on="Get position registers" class="Bool"("DisabledEnum"=w57) -> ()  [unwired: 2 in, 2 out]
    n268 = property on="Get string registers" class="Bool"("DisabledEnum"=w57) -> ()  [unwired: 2 in, 2 out]
    n269 = local read "Snpx"() -> (w55:refnum<k24>)
    n270 = call "SnpxIsConnected.vi"("Snpx"=w55) -> ("Connected"=w45:bool)  [unwired: 9 in, 1 out]
    "SNPX connected" <- w45
    n271 = Not(x=w45) -> (.not. x?=w56:bool)
    n272 = case shown="True" w45 {
      tunnel: [T12."Disabled and Grayed Out" ("Disabled") T12."Enabled" ("Disabled")] -> w44
      frame False {
      }
      frame True {
      }
    }
    n273 = case shown="True" w45 {
      tunnel: "Continuous read world position" -> [_ w158]
      tunnel: "Continuous read user frame position" -> [_ w157]
      tunnel: "Read numeric register" -> [_ w156]
      tunnel: "Write numeric register" -> [_ w155]
      tunnel: "Read string register" -> [_ w150]
      tunnel: "Write string register" -> [_ w149]
      tunnel: "Read position register" -> [_ w148]
      tunnel: "Write cartesian position register" -> [_ w147]
      tunnel: "Write joints position register" -> [_ w143]
      frame False {
      }
      frame True {
        n274 = case shown="True" w158 {
          frame False {
          }
          frame True {
            n275 = local read "Snpx"() -> (w188:refnum<k24>)
            n276 = call "GetWorldPosition.vi"("Snpx"=w188) -> ("UserTool"=→"UserTool":i16, "Cartesian position"=→"Cartesian position":T11, "JointsPosition"=→"JointsPosition":dbl[], "error out"=→"error out":errorcluster)  [unwired: 7 in]
          }
        }
        n277 = case shown="True" w157 {
          frame False {
          }
          frame True {
            n278 = local read "Snpx"() -> (w184:refnum<k24>)
            n279 = call "GetUserFramePosition.vi"("userFrame"="userFrame", "Snpx"=w184) -> ("UserTool"=→"UserTool":i16, "Cartesian position"=→"Cartesian position":T11, "error out"=→"error out 2":errorcluster)  [unwired: 6 in, 1 out]
          }
        }
        n280 = case shown="True" w150 {
          tunnel: "String register" -> [_ w175]
          frame False {
          }
          frame True {
            n281 = local read "Snpx"() -> (w176:refnum<k24>)
            n282 = call "ReadStringRegister.vi"("index"=w175, "Snpx"=w176) -> ("Value"=→"Value":string)  [unwired: 8 in, 1 out]
          }
        }
        n283 = case shown="True" w143 {
          tunnel: "Position register" -> [_ w160]
          tunnel: "Joints position" -> [_ w159]
          frame False {
          }
          frame True {
            n284 = local read "Snpx"() -> (w161:refnum<k24>)
            n285 = call "WriteJointPositionRegister.vi"("Value"=w159, "index"=w160, "Snpx"=w161) -> ()  [unwired: 8 in, 1 out]
          }
        }
        n286 = case shown="True" w148 {
          tunnel: "Position register" -> [_ w169]
          frame False {
          }
          frame True {
            n287 = local read "Snpx"() -> (w170:refnum<k24>)
            n288 = call "ReadPositionRegister.vi"("Snpx"=w170, "index"=w169) -> ("UserFrame"=→"UserFrame":i16, "Cartesian position"=w168:T10, "UserTool"=→"UserTool":i16, "Joint position"=w165:dbl[])  [unwired: 9 in, 1 out]
            n289 = property on="Cartesian position" class="Clust (strict)"("Value"=w168) -> ()  [unwired: 2 in, 2 out]
            n290 = property on="Joints position" class="Arr (strict)"("Value"=w165) -> ()  [unwired: 2 in, 2 out]
          }
        }
        n291 = case shown="True" w149 {
          tunnel: "String register" -> [_ w172]
          tunnel: "New value" -> [_ w171]
          frame False {
          }
          frame True {
            n292 = local read "Snpx"() -> (w173:refnum<k24>)
            n293 = call "WriteStringRegister.vi"("value"=w171, "index"=w172, "Snpx"=w173) -> ()  [unwired: 8 in, 1 out]
          }
        }
        n294 = case shown="True" w156 {
          tunnel: "Numeric register" -> [_ w181]
          frame False {
          }
          frame True {
            n295 = local read "Snpx"() -> (w182:refnum<k24>)
            n296 = call "ReadNumericRegister.vi"("index"=w181, "Snpx"=w182) -> ("Value"=→"Value":sgl)  [unwired: 8 in, 1 out]
          }
        }
        n297 = case shown="True" w147 {
          tunnel: "Cartesian position 2" -> [_ w163]
          tunnel: "Position register" -> [_ w162]
          frame False {
          }
          frame True {
            n298 = local read "Snpx"() -> (w164:refnum<k24>)
            n299 = call "WriteCartesianPositionRegister.vi"("Cartesian position"=w163, "index"=w162, "Snpx"=w164) -> ()  [unwired: 8 in, 1 out]
          }
        }
        n300 = case shown="True" w155 {
          tunnel: "New value" -> [_ w178]
          tunnel: "Numeric register" -> [_ w177]
          frame False {
          }
          frame True {
            n301 = local read "Snpx"() -> (w179:refnum<k24>)
            n302 = call "WriteNumericRegister.vi"("Value"=w178, "index"=w177, "Snpx"=w179) -> ()  [unwired: 8 in, 1 out]
          }
        }
      }
    }
    n303 = property on="SNPX warning" class="Str"("Visible"=w56) -> ()  [unwired: 2 in, 2 out]
    n304 = property on="Read string register" class="Bool"("DisabledEnum"=w44) -> ()  [unwired: 2 in, 2 out]
    n305 = property on="Write string register" class="Bool"("DisabledEnum"=w44) -> ()  [unwired: 2 in, 2 out]
    n306 = property on="Read numeric register" class="Bool"("DisabledEnum"=w44) -> ()  [unwired: 2 in, 2 out]
    n307 = property on="Write numeric register" class="Bool"("DisabledEnum"=w44) -> ()  [unwired: 2 in, 2 out]
    n308 = property on="Write joints position register" class="Bool"("DisabledEnum"=w44) -> ()  [unwired: 2 in, 2 out]
    n309 = property on="Continuous read user frame position" class="Bool (strict)"("DisabledEnum"=w44) -> ()  [unwired: 2 in, 2 out]
    n310 = property on="Write cartesian position register" class="Bool"("DisabledEnum"=w44) -> ()  [unwired: 2 in, 2 out]
    n311 = property on="Continuous read world position" class="Bool (strict)"("DisabledEnum"=w44) -> ()  [unwired: 2 in, 2 out]
    n312 = property on="Read position register" class="Bool"("DisabledEnum"=w44) -> ()  [unwired: 2 in, 2 out]
    n313 = local read "Cgtp"() -> (w43:refnum<k24>)
    n314 = call "CgtpIsEnabled.vi"("Cgtp"=w43) -> ("Enabled"=w37:bool)  [unwired: 9 in, 1 out]
    "CGTP Enabled" <- w37
    n315 = case shown="True" "Write variable as real" {
      tunnel: "Variable name" -> [_ w117]
      tunnel: "New real value" -> [_ w116]
      frame False {
      }
      frame True {
        n316 = local read "Cgtp"() -> (w118:refnum<k24>)
        n317 = call "CgtpWriteVariableAsReal.vi"("Cgtp"=w118, "varName"=w117, "value"=w116) -> ()  [unwired: 12 in, 1 out]
      }
    }
    n318 = case shown="True" w37 {
      tunnel: "Program name" -> [_ w129]
      tunnel: "Run" -> [_ w132]
      tunnel: "Abort" -> [_ w131]
      tunnel: "Pause" -> [_ w130]
      frame False {
      }
      frame True {
        n319 = case shown="True" w132 {
          tunnel: w129 -> [_ w137]
          frame False {
          }
          frame True {
            n320 = local read "Cgtp"() -> (w138:refnum<k24>)
            n321 = call "CgtpRunProgram.vi"("lineNum"=1, "progName"=w137, "Cgtp"=w138) -> ()  [unwired: 8 in, 1 out]
          }
        }
        n322 = case shown="True" w130 {
          frame False {
          }
          frame True {
            n323 = local read "Cgtp"() -> (w135:refnum<k24>)
            n324 = call "CgtpPauseAllPrograms.vi"("Cgtp"=w135) -> ()  [unwired: 10 in, 1 out]
          }
        }
        n325 = case shown="True" w131 {
          tunnel: w129 -> [_ w133]
          frame False {
          }
          frame True {
            n326 = local read "Cgtp"() -> (w134:refnum<k24>)
            n327 = call "CgtpAbortTask.vi"("progName"=w133, "Cgtp"=w134) -> ()  [unwired: 9 in, 1 out]
          }
        }
      }
    }
    n328 = case shown="True" "Write variable as integer" {
      tunnel: "Variable name" -> [_ w120]
      tunnel: "String value" -> [_ w119]
      frame False {
      }
      frame True {
        n329 = local read "Cgtp"() -> (w121:refnum<k24>)
        n330 = call "CgtpWriteVariableAsString.vi"("Cgtp"=w121, "varName"=w120, "value"=w119) -> ()  [unwired: 12 in, 1 out]
      }
    }
    n331 = case shown="True" "Write variable as string" {
      tunnel: "Variable name" -> [_ w123]
      tunnel: "New integer value" -> [_ w122]
      frame False {
      }
      frame True {
        n332 = local read "Cgtp"() -> (w124:refnum<k24>)
        n333 = call "CgtpWriteVariableAsInteger.vi"("Cgtp"=w124, "varName"=w123, "value"=w122) -> ()  [unwired: 12 in, 1 out]
      }
    }
    n334 = case shown="True" "Read variable" {
      tunnel: "Variable name" -> [_ w127]
      frame False {
      }
      frame True {
        n335 = local read "Cgtp"() -> (w128:refnum<k24>)
        n336 = call "CgtpReadVariableAsString.vi"("varName"=w127, "Cgtp"=w128) -> ("String Value"=w126:string, "error out"=w125:errorcluster)  [unwired: 8 in]
        n337 = property on="String value" class="Str"(error in=w125, "Value"=w126) -> ()  [unwired: 1 in, 2 out]
      }
    }
    n338 = Not(x=w37) -> (.not. x?=w36:bool)
    n339 = case shown="True" w37 {
      tunnel: [T12."Disabled and Grayed Out" ("Disabled") T12."Enabled" ("Disabled")] -> w42
      frame False {
      }
      frame True {
      }
    }
    n340 = property on="CGTP warning" class="Str"("Visible"=w36) -> ()  [unwired: 2 in, 2 out]
    n341 = property on="Pause" class="Bool"("DisabledEnum"=w42) -> ()  [unwired: 2 in, 2 out]
    n342 = property on="Abort" class="Bool"("DisabledEnum"=w42) -> ()  [unwired: 2 in, 2 out]
    n343 = property on="Run" class="Bool"("DisabledEnum"=w42) -> ()  [unwired: 2 in, 2 out]
  }
  "TelnetError" <- "" ("ErrorText")
  "TelnetSucceed" <- FALSE ("Succeed")
  "KclCommand" <- "" ("KclCommand")
  "Telnet warning" <- "Telnet is not connected\nPlease connect to use this panel" ("Telnet warning")
  "FTP warning" <- "FTP is not connected\nPlease connect to use this panel" ("FTP warning")
  "SNPX warning" <- "SNPX is not connected\nPlease connect to use this panel" ("FTP warning")
  "CGTP warning" <- "CGTP is not connected\nPlease connect to use this panel" ("Telnet warning 2")
